vi "Calculate Contour Vertices.vi"(7 "Contour Property In":T2={"Contour Type"=enum."Contour with surface", "Axis Basis"=enum."X-Axis", "Level List"=[], "Level Mode"=enum."Levels", "Levels"=0, "Interval"=0.0}, 9 "Range In":T1, 10 "Mesh Index Array":u32[](array[numeric]), 11 "Mesh Vertex Array In":cluster{"X":sgl, "Y":sgl, "Z":sgl}[](array[cluster])) -> (1 "Range Out":T1, 3 "Contour Vertex Array Out":cluster{"X":sgl, "Y":sgl, "Z":sgl}[](array[cluster]))   [LabVIEW 2020, in "3D Contour.lvclass"]
uses:
  <vilib>/Math Plots/3D Math Plots/3D Contour/3D Contour/3D Contour.lvclass
  <vilib>/Math Plots/3D Math Plots/3D Plot/3D Plot/Typedef/Range Clusters.ctl
  <vilib>/Math Plots/3D Math Plots/3D Plot/3D Plot/3D Plot.lvclass
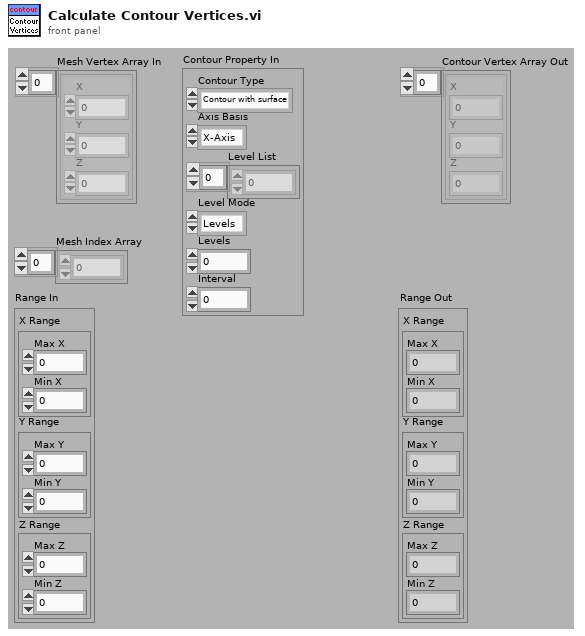
[diagram p1: front panel]
types:
  T1 = typedef "3D Plot.lvclass/Range Clusters.ctl" = cluster{"X Range":cluster{"Max X":sgl, "Min X":sgl}, "Y Range":cluster{"Max Y":sgl, "Min Y":sgl}, "Z Range":cluster{"Max Z":sgl, "Min Z":sgl}}
  T2 = cluster{"Contour Type":enum16{"Contour", "Contour with surface"}, "Axis Basis":enum16{"X-Axis", "Y-Axis", "Z-Axis"}, "Level List":sgl[], "Level Mode":enum16{"Levels", "Interval", "Level List"}, "Levels":u16, "Interval":sgl}
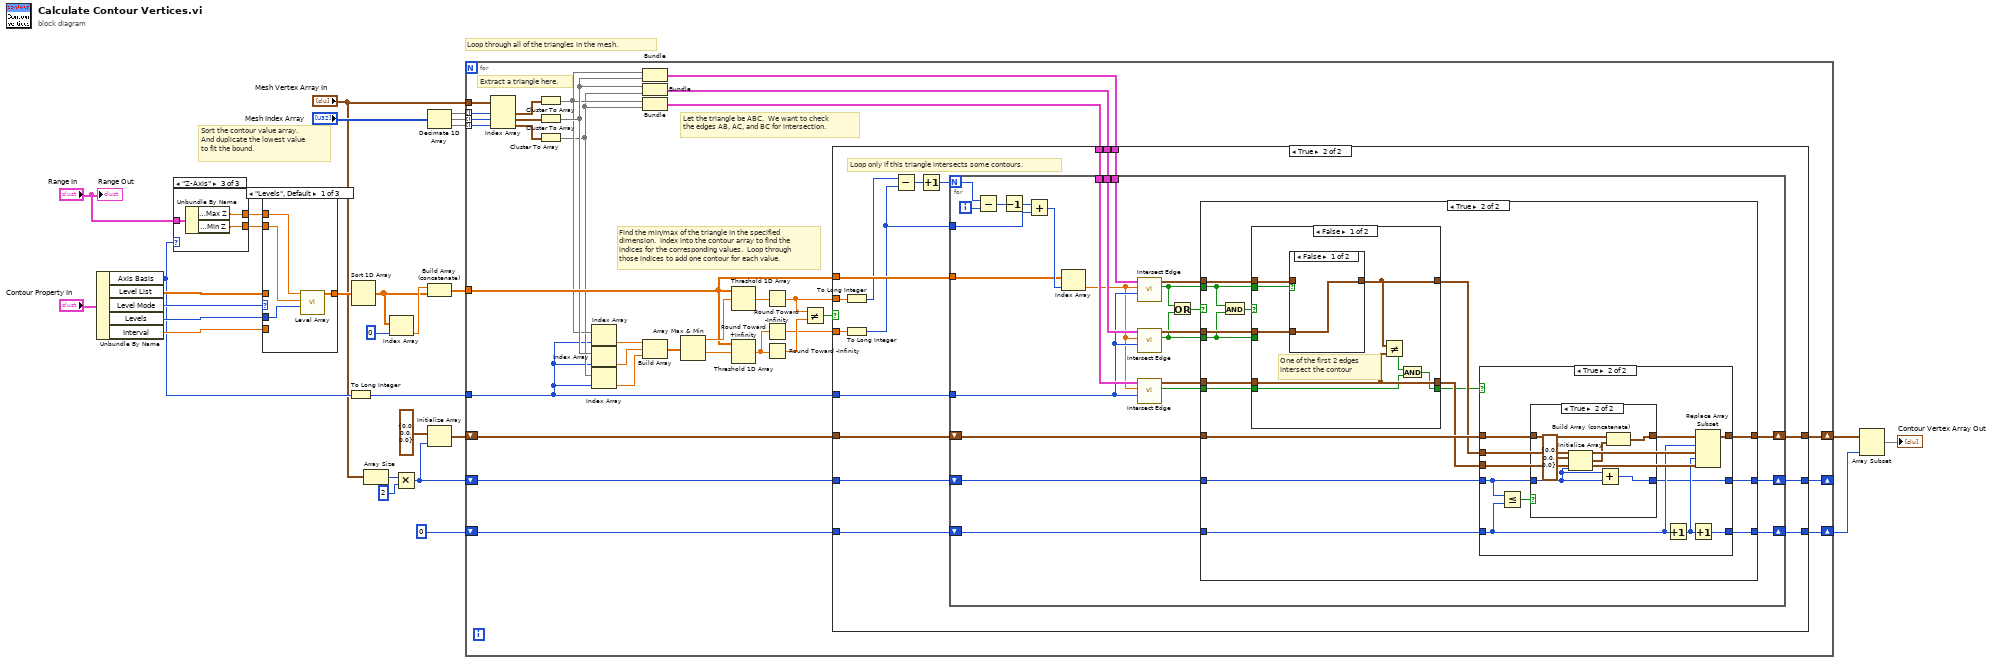
[diagram p0: block diagram]
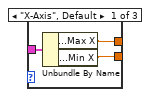
[diagram p2: hidden frame]
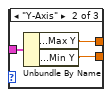
[diagram p3: hidden frame]
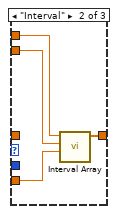
[diagram p4: hidden frame]
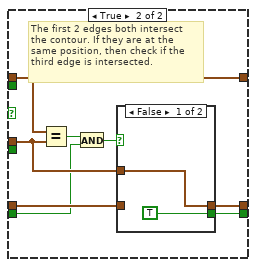
[diagram p11: hidden frame]
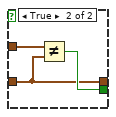
[diagram p12: hidden frame]
diagram:
  # "Sort the contour value array.\nAnd duplicate the lowest value\nto fit the bound."
  # "Loop through all of the triangles in the mesh."
  n1 = Unbundle By Name("Contour Property In") -> ("Axis Basis"=w16:enum16{"X-Axis", "Y-Axis", "Z-Axis"}, "Level List"=w19:sgl[], "Level Mode"=w21:enum16{"Levels", "Interval", "Level List"}, "Levels"=w18:u16, "Interval"=w17:sgl)
  n2 = case shown="\"Z-Axis\"" w16 {
    tunnel: "Range In" -> [w32 w35 w38]
    tunnel: [w31 w34 w37] -> w15
    tunnel: [w30 w33 w36] -> w14
    frame "X-Axis", Default {
      n3 = Unbundle By Name(w32) -> ("X Range.Max X"=w31:sgl, "X Range.Min X"=w30:sgl)
    }
    frame "Y-Axis" {
      n4 = Unbundle By Name(w35) -> ("Y Range.Max Y"=w34:sgl, "Y Range.Min Y"=w33:sgl)
    }
    frame "Z-Axis" {
      n5 = Unbundle By Name(w38) -> ("Z Range.Max Z"=w37:sgl, "Z Range.Min Z"=w36:sgl)
    }
  }
  n6 = case shown="\"Levels\", Default" w21 {
    tunnel: [w42 w46 w47] -> w20
    tunnel: w19 -> [_ _ w47]
    tunnel: w18 -> [w41 _ _]
    tunnel: w17 -> [_ w45 _]
    tunnel: w15 -> [w40 w44 _]
    tunnel: w14 -> [w39 w43 _]
    frame "Levels", Default {
      n7 = call <vilib>:"Level Array.vi"("Level"=w41, "Min"=w39, "Max"=w40) -> ("Level Array"=w42:sgl[])  [unwired: 8 out]
    }
    frame "Interval" {
      n8 = call <vilib>:"Interval Array.vi"("Interval"=w45, "Min"=w43, "Max"=w44) -> ("Level Array"=w46:sgl[])  [unwired: 8 out]
    }
    frame "Level List" {
    }
  }
  n9 = To Long Integer(number=w16) -> (32bit integer=w13:i32)
  n10 = Sort 1D Array(array=w20) -> (sorted array=w23:sgl[])
  n11 = Array Size(array="Mesh Vertex Array In") -> (size(s)=w6:i32)
  n12 = Index Array(array=w23, index=0) -> (element=w24:sgl)
  n13 = Multiply(x=w6, y=2) -> (x*y=w5:i32)
  n14 = Decimate 1D Array("Mesh Index Array") -> (w28:u32[], w25:u32[], w26:u32[])
  n15 = Build Array (concatenate)(w24, w23) -> (w22:sgl[])
  n16 = Initialize Array(cluster{"X":sgl, "Y":sgl, "Z":sgl} {"X"=0.0, "Y"=0.0, "Z"=0.0} ("3D Point 2"), w5) -> (w9:cluster{"X":sgl, "Y":sgl, "Z":sgl}[])
  n17 = for {
    tunnel: w22 -> [w70]
    tunnel: w28 -> [w62] mode=indexing
    tunnel: w25 -> [w61] mode=indexing
    tunnel: w26 -> [w60] mode=indexing
    tunnel: "Mesh Vertex Array In" -> [w63]
    tunnel: w13 -> [w54]
    shift-right: [w52] -> w3
    shift-left: w9 -> [w53]
    shift-right: [w49] -> w1
    shift-left: 0 ("index") -> [w51]
    shift-right: [w48] -> _
    shift-left: w5 -> [w50]
    # "Find the min/max of the triangle in the specified dimension.  Index into the contour array to find the indices for the corresponding values.  Loop through those indices to add one contour for each value."
    # "Let the triangle be ABC.  We want to check the edges AB, AC, and BC for intersection."
    # "Extract a triangle here."
    n18 = Index Array(array=w63, index #1=w62, index #2=w61, index #3=w60) -> (element #1=w59:cluster{"X":sgl, "Y":sgl, "Z":sgl}, element #2=w58:cluster{"X":sgl, "Y":sgl, "Z":sgl}, element #3=w57:cluster{"X":sgl, "Y":sgl, "Z":sgl})
    n19 = Cluster To Array(cluster=w59) -> (array=w68:sgl[])
    n20 = Cluster To Array(cluster=w58) -> (array=w69:sgl[])
    n21 = Cluster To Array(cluster=w57) -> (array=w64:sgl[])
    n22 = Index Array(array=w68, index=w54) -> (element=w80:sgl)
    n23 = Index Array(array=w69, index=w54) -> (element=w79:sgl)
    n24 = Index Array(array=w64, index=w54) -> (element=w78:sgl)
    n25 = Bundle("3D Point 2"=w68, "3D Point 2"=w69) -> (w67:cluster{"3D Point 2":sgl[], "3D Point 2":sgl[]})  [unwired: 1 out]
    n26 = Bundle("3D Point 2"=w69, "3D Point 2"=w64) -> (w66:cluster{"3D Point 2":sgl[], "3D Point 2":sgl[]})  [unwired: 1 out]
    n27 = Bundle("3D Point 2"=w68, "3D Point 2"=w64) -> (w65:cluster{"3D Point 2":sgl[], "3D Point 2":sgl[]})  [unwired: 1 out]
    n28 = Build Array(w80, w79, w78) -> (w77:sgl[])
    n29 = Array Max & Min(array=w77) -> (max value=w76:sgl, min value=w75:sgl)  [unwired: 2 out]
    n30 = Threshold 1D Array(2:w76, 3:w70) -> (0:w55:sgl)  [unwired: 1 out]
    n31 = Threshold 1D Array(2:w75, 3:w70) -> (0:w56:sgl)  [unwired: 1 out]
    n32 = Round Toward -Infinity(1:w55) -> (0:w71:sgl)
    n33 = Round Toward +Infinity(x=w56) -> (ceil(x): smallest int >= x=w72:sgl)
    n34 = Round Toward -Infinity(1:w56) -> (0:w74:sgl)
    n35 = Not Equal?(x=w71, y=w74) -> (x != y?=w73:bool)
    n36 = case shown="True" w73 {
      tunnel: w72 -> [_ w92]
      tunnel: w71 -> [_ w93]
      tunnel: w70 -> [_ w98]
      tunnel: w67 -> [_ w97]
      tunnel: w66 -> [_ w96]
      tunnel: w65 -> [_ w95]
      tunnel: w54 -> [_ w94]
      tunnel: w53 -> [w83 w89]
      tunnel: [w83 w88] -> w52
      tunnel: w51 -> [w81 w87]
      tunnel: w50 -> [w82 w86]
      tunnel: [w81 w85] -> w49
      tunnel: [w82 w84] -> w48
      frame False {
        # "The triangle does not intersect any contours."
      }
      frame True {
        # "Loop only if this triangle intersects some contours."
        n37 = To Long Integer(number=w93) -> (32bit integer=w90:i32)
        n38 = To Long Integer(number=w92) -> (32bit integer=w91:i32)
        n39 = Subtract(x=w90, y=w91) -> (x-y=w100:i32)
        n40 = Increment(x=w100) -> (x+1=w99:i32)
        n41 = for {
          N: w99 -> [w125]
          tunnel: w91 -> [w120]
          tunnel: w98 -> [w119]
          tunnel: w97 -> [w118]
          tunnel: w96 -> [w117]
          tunnel: w95 -> [w116]
          tunnel: w94 -> [w115]
          shift-right: [w109] -> w88
          shift-left: w89 -> [w110]
          shift-right: [w102] -> w85
          shift-left: w87 -> [w104]
          shift-right: [w101] -> w84
          shift-left: w86 -> [w103]
          i -> [w124]
          n42 = Subtract(x=w125, y=w124) -> (x-y=w123:i32)
          n43 = Decrement(x=w123) -> (x-1=w122:i32)
          n44 = Add(x=w122, y=w120) -> (x+y=w121:i32)
          n45 = Index Array(array=w119, index=w121) -> (element=w114:sgl)
          n46 = call <vilib>:"Intersect Edge.vi"("Axis Basis"=w115, "Contour Value"=w114, "Triangle Array Cluster"=w118) -> ("In Range"=w107:bool, "Intersect Point"=w113:cluster{"X":sgl, "Y":sgl, "Z":sgl})  [unwired: 7 out]
          n47 = call <vilib>:"Intersect Edge.vi"("Axis Basis"=w115, "Contour Value"=w114, "Triangle Array Cluster"=w117) -> ("In Range"=w106:bool, "Intersect Point"=w112:cluster{"X":sgl, "Y":sgl, "Z":sgl})  [unwired: 7 out]
          n48 = call <vilib>:"Intersect Edge.vi"("Axis Basis"=w115, "Contour Value"=w114, "Triangle Array Cluster"=w116) -> ("In Range"=w105:bool, "Intersect Point"=w111:cluster{"X":sgl, "Y":sgl, "Z":sgl})  [unwired: 7 out]
          n49 = Or(x=w107, y=w106) -> (x .or. y?=w108:bool)
          n50 = case shown="True" w108 {
            tunnel: w113 -> [_ w144]
            tunnel: w112 -> [_ w143]
            tunnel: w111 -> [_ w142]
            tunnel: w107 -> [_ w140]
            tunnel: w106 -> [_ w139]
            tunnel: w110 -> [w128 w137]
            tunnel: [w128 w136] -> w109
            tunnel: w105 -> [_ w138]
            tunnel: w104 -> [w126 w132]
            tunnel: w103 -> [w127 w131]
            tunnel: [w126 w130] -> w102
            tunnel: [w127 w129] -> w101
            frame False {
              # "This case has no contour line encounter. \n\nTo form a line, there should be at least 2 vertices.\nThe first 2 edges do not intersect the contour, \nthen the third edge also do not intersect."
            }
            frame True {
              n51 = And(x=w140, y=w139) -> (x .and. y?=w141:bool)
              n52 = case shown="False" w141 {
                tunnel: w144 -> [w173 w180]
                tunnel: w143 -> [w172 w184]
                tunnel: w142 -> [w170 w183]
                tunnel: w140 -> [w174 _]
                tunnel: w139 -> [_ _]
                tunnel: w138 -> [w168 w182]
                tunnel: [w171 w180] -> w135
                tunnel: [w170 w179] -> w134
                tunnel: [w167 w177] -> w133
                frame False {
                  # "One of the first 2 edges \nintersect the contour"
                  n53 = case shown="False" w174 {
                    tunnel: [w175 w176] -> w171
                    tunnel: w173 -> [_ w176]
                    tunnel: w172 -> [w175 _]
                    frame False {
                    }
                    frame True {
                    }
                  }
                  n54 = Not Equal?(x=w171, y=w170) -> (x != y?=w169:bool)
                  n55 = And(x=w169, y=w168) -> (x .and. y?=w167:bool)
                }
                frame True {
                  # "The first 2 edges both intersect \nthe contour. If they are at the \nsame position, then check if the \nthird edge is intersected."
                  n56 = Equal?(x=w180, y=w184) -> (x = y?=w178:bool)
                  n57 = And(x=w178, y=w182) -> (x .and. y?=w181:bool)
                  n58 = case shown="False" w181 {
                    tunnel: w184 -> [w186 w188]
                    tunnel: w183 -> [_ w187]
                    tunnel: [w186 w187] -> w179
                    tunnel: [TRUE ("In Range") w189] -> w177
                    frame False {
                    }
                    frame True {
                      n59 = Not Equal?(x=w188, y=w187) -> (x != y?=w189:bool)
                    }
                  }
                }
              }
              n60 = case shown="True" w133 {
                tunnel: w137 -> [w147 w151]
                tunnel: [w147 w158] -> w136
                tunnel: w135 -> [_ w157]
                tunnel: w134 -> [_ w156]
                tunnel: w132 -> [w145 w153]
                tunnel: w131 -> [w146 w149]
                tunnel: [w145 w154] -> w130
                tunnel: [w146 w148] -> w129
                frame False {
                  # "If they are at \nsame position,\nignore them"
                }
                frame True {
                  n61 = Less Or Equal?(x=w149, y=w153) -> (x <= y?=w152:bool)
                  n62 = case shown="True" w152 {
                    tunnel: w151 -> [w160 w164]
                    tunnel: [w160 w163] -> w150
                    tunnel: w149 -> [w159 w162]
                    tunnel: [w159 w161] -> w148
                    frame False {
                    }
                    frame True {
                      n63 = Initialize Array(cluster{"X":sgl, "Y":sgl, "Z":sgl} {"X"=0.0, "Y"=0.0, "Z"=0.0} ("3D Point 2"), w162) -> (w165:cluster{"X":sgl, "Y":sgl, "Z":sgl}[])
                      n64 = Add(x=w162, y=w162) -> (x+y=w161:i32)
                      n65 = Build Array (concatenate)(w164, w165) -> (w163:cluster{"X":sgl, "Y":sgl, "Z":sgl}[])
                    }
                  }
                  n66 = Increment(x=w153) -> (x+1=w155:i32)
                  n67 = Increment(x=w155) -> (x+1=w154:i32)
                  n68 = Replace Array Subset(array=w150, new element #1=w157, index #1=w153, new element #2=w156, index #2=w155) -> (w158:cluster{"X":sgl, "Y":sgl, "Z":sgl}[])
                }
              }
            }
          }
        }
      }
    }
  }
  n69 = Array Subset(array=w3, length=w1) -> (→"Contour Vertex Array Out":cluster{"X":sgl, "Y":sgl, "Z":sgl}[])  [unwired: 1 in]
  "Range Out" <- "Range In"
